vi "Ball Counter.vi"   [LabVIEW 2025]
uses:
  Globals.vi
  <vilib>/Rock Robotics/Network Tables/NT Write Integer.vi
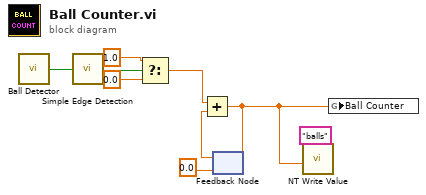
[diagram p0: block diagram]
diagram:
  n1 = call "Ball Detector.vi"() -> ("Has Balls?"=w9:bool)  [unwired: 3 in]
  n2 = call "Simple Edge Detection.vi"("In"=w9) -> ("Rising Edge"=w8:bool)  [unwired: 1 out]
  n3 = Select(t=1.0, s=w8, f=0.0) -> (s? t:f=w5:dbl)
  n4 = feedback #1(0.0) -> (w4:dbl)
  n5 = Add(x=w5, y=w4) -> (x+y=w1:dbl)
  n6 = feedback-in #1(w1) -> ()
  n7 = call-poly <vilib>:"NT Write Value.vi"("value"=w1, "name"="balls") -> ()  [unwired: 9 in, 1 out]
  n8 = global write "Globals.vi" "Ball Counter"(w1) -> ()
